vi "RandomHeightmap.vi"(10 "y":i32, 11 "x":i32) -> (3 "Array":dbl[][](array[numeric]))   [LabVIEW 2016]
panel:
  in  "zmult":dbl
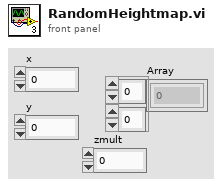
[diagram p1: front panel]
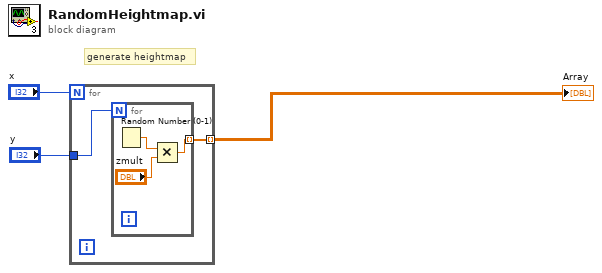
[diagram p0: block diagram]
diagram:
  # "generate heightmap"
  n1 = for {
    N: "x" -> [_]
    tunnel: [w5] -> w2 mode=indexing
    tunnel: "y" -> [w4]
    n2 = for {
      N: w4 -> [_]
      tunnel: [w6] -> w5 mode=indexing
      n3 = Random Number (0-1)() -> (number: 0 to 1=w7:dbl)
      n4 = Multiply(x=w7, y="zmult") -> (x*y=w6:dbl)
    }
  }
  "Array" <- w2
